vi "Samsung RTP Test.vi"() -> ()   [LabVIEW 2014]
uses:
  <userlib>/cRIO Master Files/Controls/NamedError.ctl
  Controls/ES String Array.ctl
  Controls/ES String Data.ctl
  Controls/ES System Data.ctl
  Controls/StringSelector.ctl
  Controls/Current Limit Parameters.ctl
panel:
  in  "Clear Error":bool
  in  "stop":bool
  out "Current Limit Parameters":T1={"Max Cell Voltage Max Setpoint"=4.1, "Max Cell Voltage Actual Value"=0.0, "Max Cell Voltage Derate Setpoint"=3.8, "Max Charge Current"=-0.0, "Min Cell Voltage Min Setpoint"=3.0, "Min Cell Voltage Actual Value"=0.0, "Min Cell Voltage Derate Setpoint"=3.3, "Max Discharge Current"=0.0} {"Min Cell Voltage Actual Value" format="%#.2f"; "Max Cell Voltage Actual Value" format="%#.2f"}
  out "ES System Data":T2={"Voltage"=0.0, "Current"=0.0, "SOC Avg"=nan, "Faults"=8192, "Alarms"=4096, "# Strings"=0, "Max Temp"=0, "Min Temp"=0, "Max Cell Voltage"=0.0, "Min Cell Voltage"=0.0, "Energy Capacity"=0.0, "Energy Remaining"=0.0, "SOC Min"=0.0, "SOC Max"=0.0, "ES Fault"=TRUE, "String Select"=enum."1 String (1)", "ES Com Fault"=FALSE, "SOH Avg"=nan}
  out "ES String Data":T4=[{"Voltage"=0.0, "State of Charge"=0.0, "Current"=0.0, "Temperature Min"=0, "Temperature Max"=0, "Faults"=8192, "Alarms"=0, "String Number"=1, "Contactor Status"=FALSE, "String Ready"=FALSE, "Fuse Status"=FALSE, "Cell V Max"=0.0, "Cell V Min"=0.0, "State of Health"=0.0}, {"Voltage"=0.0, "State of Charge"=0.0, "Current"=0.0, "Temperature Min"=0, "Temperature Max"=0, "Faults"=8192, "Alarms"=0, "String Number"=2, "Contactor Status"=FALSE, "String Ready"=FALSE, "Fuse Status"=FALSE, "Cell V Max"=0.0, "Cell V Min"=0.0, "State of Health"=0.0}, {"Voltage"=0.0, "State of Charge"=0.0, "Current"=0.0, "Temperature Min"=0, "Temperature Max"=0, "Faults"=8192, "Alarms"=0, "String Number"=3, "Contactor Status"=FALSE, "String Ready"=FALSE, "Fuse Status"=FALSE, "Cell V Max"=0.0, "Cell V Min"=0.0, "State of Health"=0.0}, {"Voltage"=0.0, "State of Charge"=0.0, "Current"=0.0, "Temperature Min"=0, "Temperature Max"=0, "Faults"=8192, "Alarms"=0, "String Number"=4, "Contactor Status"=FALSE, "String Ready"=FALSE, "Fuse Status"=FALSE, "Cell V Max"=0.0, "Cell V Min"=0.0, "State of Health"=0.0}, {"Voltage"=0.0, "State of Charge"=0.0, "Current"=0.0, "Temperature Min"=0, "Temperature Max"=0, "Faults"=8192, "Alarms"=0, "String Number"=5, "Contactor Status"=FALSE, "String Ready"=FALSE, "Fuse Status"=FALSE, "Cell V Max"=0.0, "Cell V Min"=0.0, "State of Health"=0.0}, {"Voltage"=0.0, "State of Charge"=0.0, "Current"=0.0, "Temperature Min"=0, "Temperature Max"=0, "Faults"=8192, "Alarms"=0, "String Number"=6, "Contactor Status"=FALSE, "String Ready"=FALSE, "Fuse Status"=FALSE, "Cell V Max"=0.0, "Cell V Min"=0.0, "State of Health"=0.0}, {"Voltage"=0.0, "State of Charge"=0.0, "Current"=0.0, "Temperature Min"=0, "Temperature Max"=0, "Faults"=8192, "Alarms"=0, "String Number"=7, "Contactor Status"=FALSE, "String Ready"=FALSE, "Fuse Status"=FALSE, "Cell V Max"=0.0, "Cell V Min"=0.0, "State of Health"=0.0}, {"Voltage"=0.0, "State of Charge"=0.0, "Current"=0.0, "Temperature Min"=0, "Temperature Max"=0, "Faults"=8192, "Alarms"=0, "String Number"=8, "Contactor Status"=FALSE, "String Ready"=FALSE, "Fuse Status"=FALSE, "Cell V Max"=0.0, "Cell V Min"=0.0, "State of Health"=0.0}, {"Voltage"=0.0, "State of Charge"=0.0, "Current"=0.0, "Temperature Min"=0, "Temperature Max"=0, "Faults"=8192, "Alarms"=0, "String Number"=9, "Contactor Status"=FALSE, "String Ready"=FALSE, "Fuse Status"=FALSE, "Cell V Max"=0.0, "Cell V Min"=0.0, "State of Health"=0.0}, {"Voltage"=0.0, "State of Charge"=0.0, "Current"=0.0, "Temperature Min"=0, "Temperature Max"=0, "Faults"=8192, "Alarms"=0, "String Number"=10, "Contactor Status"=FALSE, "String Ready"=FALSE, "Fuse Status"=FALSE, "Cell V Max"=0.0, "Cell V Min"=0.0, "State of Health"=0.0}]
  in  "ES ON Array":bool[](array[boolean])=[FALSE, FALSE, FALSE, FALSE, FALSE, FALSE, FALSE, FALSE, FALSE, FALSE]
  out "ES Error":T6={"status"=FALSE, "code"=0, "source"="", "Name"="ES Comms"}
  out "ES Count":i32=15
  out "Contactor CMD FB":bool[](array[boolean])
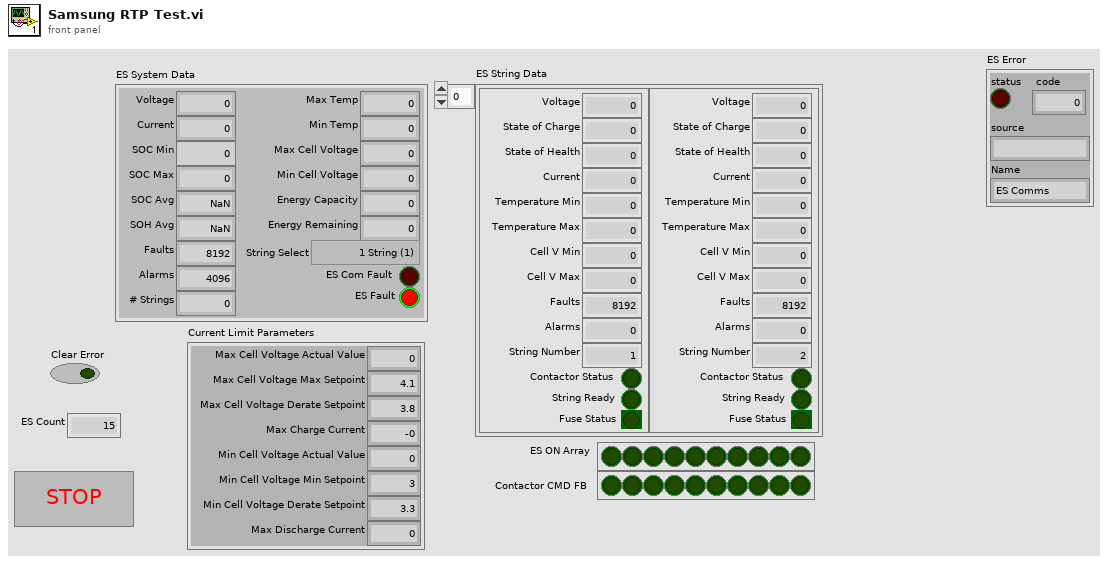
[diagram p1: front panel]
types:
  T1 = typedef "Current Limit Parameters.ctl" = cluster{"Max Cell Voltage Max Setpoint":dbl, "Max Cell Voltage Actual Value":dbl, "Max Cell Voltage Derate Setpoint":dbl, "Max Charge Current":dbl, "Min Cell Voltage Min Setpoint":dbl, "Min Cell Voltage Actual Value":dbl, "Min Cell Voltage Derate Setpoint":dbl, "Max Discharge Current":dbl}
  T2 = typedef "ES System Data.ctl" = cluster{"Voltage":sgl, "Current":sgl, "SOC Avg":sgl, "Faults":u16, "Alarms":u16, "# Strings":u16, "Max Temp":i16, "Min Temp":i16, "Max Cell Voltage":sgl, "Min Cell Voltage":sgl, "Energy Capacity":sgl, "Energy Remaining":sgl, "SOC Min":sgl, "SOC Max":sgl, "ES Fault":bool, "String Select":T3, "ES Com Fault":bool, "SOH Avg":sgl}
  T3 = typedef "StringSelector.ctl" = enum16{"1 String (1)", "1 String (2)", "1 String (3)", "2 Strings (1 2)", "2 Strings (2 3)", "2 Strings (1 3)", "3 Strings"}
  T4 = typedef "ES String Array.ctl" = T5[]
  T5 = typedef "ES String Data.ctl" = cluster{"Voltage":sgl, "State of Charge":sgl, "Current":sgl, "Temperature Min":i16, "Temperature Max":i16, "Faults":u16, "Alarms":u16, "String Number":u16, "Contactor Status":bool, "String Ready":bool, "Fuse Status":bool, "Cell V Max":dbl, "Cell V Min":dbl, "State of Health":sgl}
  T6 = typedef "NamedError.ctl" = cluster{"status":bool, "code":i32, "source":string, "Name":string}
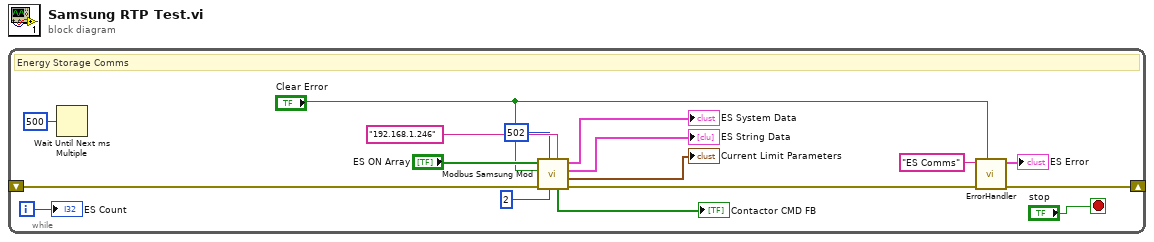
[diagram p0: block diagram]
diagram:
  n1 = while "Energy Storage Comms" {
    shift-right: [w15] -> _
    shift-left: _ -> [w3]
    i -> [w8]
    stop <- "stop" stop-if-true
    # "Energy Storage Comms"
    n2 = Wait Until Next ms Multiple(millisecond multiple=u32 500 ("milliseconds to wait")) -> ()  [unwired: 1 out]
    n3 = call "Modbus Samsung Mod.vi"("address"="192.168.1.246", "# Racks"=2, "port (502)"=u16 502, "Error In"=w3, "ES Reset"="Clear Error", "ES ON Array"="ES ON Array") -> ("Error Out"=w16:errorcluster, "Current Limit Parameters Out"=→"Current Limit Parameters":T1, "Energy Storage String Data Out"=→"ES String Data":T4, "Energy Storage System Data Out"=→"ES System Data":T2, "Contactor CMD FB"=→"Contactor CMD FB":bool[])  [unwired: 1 in]
    n4 = call <userlib>:"ErrorHandler.vi"("Clear Error"="Clear Error", "Error In"=w16, "Name"="ES Comms") -> ("Error Out"=w15:errorcluster, "Named Error Out"=→"ES Error":T6)  [unwired: 5 in]
    "ES Count" <- w8
  }
